vi "recycle_.vi"(8 "error in (no error)":errorcluster, 9 "Position":T1, 10 "recycle room":string) -> (0 "error out":errorcluster, 1 "Position out":T1)   [LabVIEW 2019]
uses:
  subVI/move/position cluster.ctl
  route_name.ctl
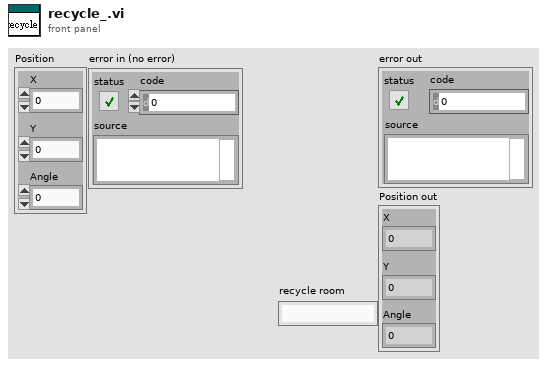
[diagram p1: front panel]
types:
  T1 = typedef "position cluster.ctl" = cluster{"X":dbl, "Y":dbl, "Angle":dbl}
  T2 = typedef "route_name.ctl" = enum16{"S-Vision", "Vision-R1", "Vision-R2", "Vision-R3", "Vision-R4", "Vision-R5", "R1-Vision", "R2-Vision", "R3-Vision", "R4-Vision", "R5-Vision", "Vision-box", "box-recycle", "recycle-box", "box-Vision", "Vision-S"}
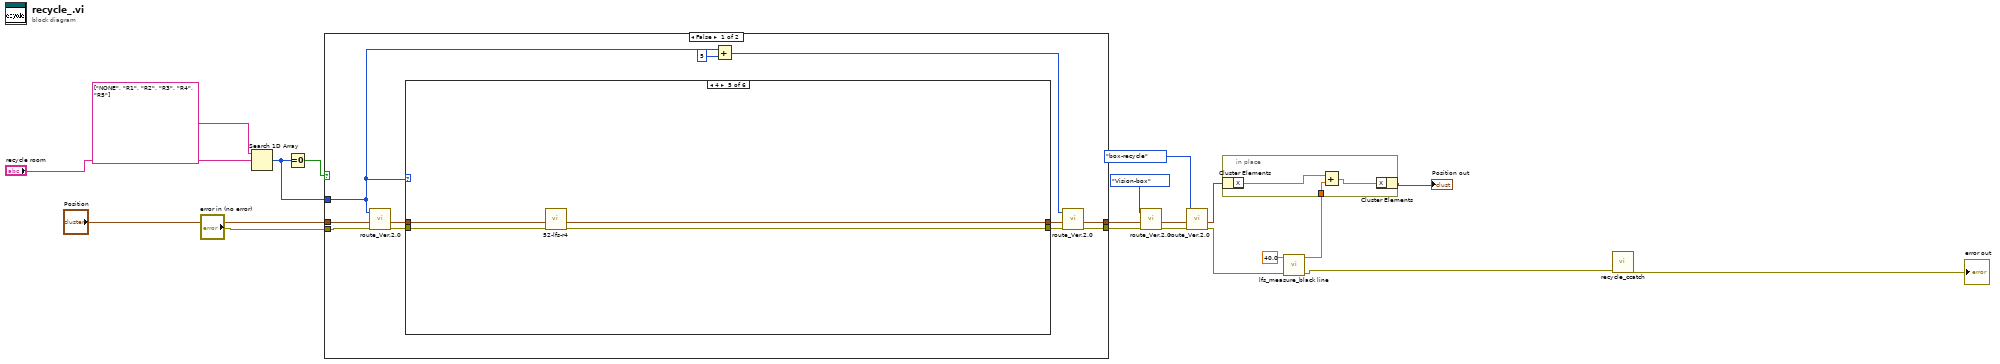
[diagram p0: block diagram]
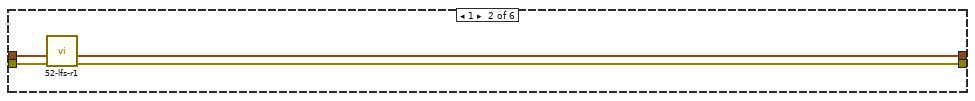
[diagram p3: hidden frame]
diagram:
  n1 = Search 1D Array(1D array=string[] ["NONE", "R1", "R2", "R3", "R4", "R5"], element="recycle room") -> (index of element=w16:i32)  [unwired: 1 in]
  n2 = Equal To 0?(x=w16) -> (x = 0?=w17:bool)
  n3 = case shown="False" w17 {
    tunnel: w16 -> [w22 _]
    tunnel: "Position" -> [w30 w48]
    tunnel: "error in (no error)" -> [w29 w47]
    tunnel: [w28 w47] -> w13
    tunnel: [w27 w48] -> w12
    frame False {
      n4 = call "route_Ver.2.0.vi"("error in (no error)"=w29, "Position"=w30, 11:w22) -> ("error out"=w26:errorcluster, "Position out"=w25:T1)  [unwired: 7 in]
      n5 = case shown="4" w22 {
        tunnel: w26 -> [w31 w36 w38 w40 w44 w46]
        tunnel: w25 -> [w32 w35 w37 w39 w43 w45]
        tunnel: [w31 w33 w38 w40 w42 w46] -> w24
        tunnel: [w32 w34 w37 w39 w41 w45] -> w23
        frame 0, Default {
        }
        frame 1 {
          n6 = call "52-lfs-r1.vi"("error in (no error)"=w36, "Position in"=w35) -> ("error out"=w33:errorcluster, "Position out"=w34:T1)  [unwired: 8 in]
        }
        frame 2 {
        }
        frame 3 {
        }
        frame 4 {
          n7 = call "52-lfs-r4.vi"("error in (no error)"=w44, "Position in"=w43) -> ("error out"=w42:errorcluster, "Position out"=w41:T1)  [unwired: 8 in]
        }
        frame 5 {
        }
      }
      n8 = Add(x=w22, y=5) -> (x+y=w20:i32)
      n9 = call "route_Ver.2.0.vi"("error in (no error)"=w24, "Position"=w23, 11:w20) -> ("error out"=w28:errorcluster, "Position out"=w27:T1)  [unwired: 7 in]
    }
    frame True {
    }
  }
  n10 = call "route_Ver.2.0.vi"("error in (no error)"=w13, "Position"=w12, 11:route_name."Vision-box") -> ("error out"=w9:errorcluster, "Position out"=w8:T1)  [unwired: 7 in]
  n11 = call "route_Ver.2.0.vi"("error in (no error)"=w9, "Position"=w8, 11:route_name."box-recycle") -> ("error out"=w4:errorcluster, "Position out"=w5:T1)  [unwired: 7 in]
  n12 = call "lfs_measure_black line.vi"("error in (no error)"=w4, "limit"=40.0) -> ("error out"=w3:errorcluster, "move cm"=w6:dbl)  [unwired: 7 in, 1 out]
  n13 = in-place {
    in-place-border: w6 -> [w50]
    n14 = in-place-cluster #1(w5) -> ("X"=w51:dbl)
    n15 = Add(x=w51, y=w50) -> (x+y=w49:dbl)
    n16 = in-place-cluster #1("X"=w49) -> (→"Position out":T1)
  }
  n17 = call "recycle_ccatch.vi"("error in (no error)"=w3) -> ("error out"=→"error out":errorcluster)  [unwired: 10 in]
